vi "Voice Enhancement.vi"() -> ()   [LabVIEW 2023]
doc: "This example shows the application of linear Time Frequency Analysis VIs in online voice enhancement, or noise reduction in speech signals. Refer to the Online Noise Reduction example for more information about online noise reduction.\n\nThis example uses the TFA Online Gabor Transform VI to convert a speech signal into the time-frequency representation, sets the Gabor coefficients whose magnitude is smaller than a threshold to zero, and finally uses the TFA Online Gabor Expansion VI to reconstruct the enhanced speech signal. \n\n<b>Instructions:</b>\n1) Run this VI.\n2) Speak into the microphone in a noisy environment.\n3) Listen the enhanced voice by using the headset."
uses:
  <vilib>/sound2/lvsound2.llb/Sound Data Format.ctl
  <vilib>/sound2/lvsound2.llb/Sound Input Read (DBL).vi
  <vilib>/addons/Time Frequency Analysis/Transform.llb/TFA Online Gabor Transform (Real).vi
  <vilib>/addons/Time Frequency Analysis/Transform.llb/TFA Online Gabor Expansion (Real).vi
  <vilib>/sound2/lvsound2.llb/Sound Output Write (DBL Single).vi
  <vilib>/addons/_Advanced Signal Processing/NI_AdvSigProcTFA.lvlib
panel:
  out "aspt-left-top":bool
  in  "Replay?(F)":bool
  in  "Attenuation factor":dbl=0.2
  in  "reset":bool
  out "Enhanced Speech":dbl[](graph)
  out "Noise Speech":dbl[](graph)
  out "Enhanced Gabor Coefficients":dbl[][](graph)
  out "Magnitude of Gabor Coefficients":dbl[][](graph)
  in  "Enhance?":bool=TRUE
  in  "Noise level":dbl=1.2
  in  "Stop":bool
  # "Overview: Shows the application of linear Time Frequency Analysis VIs in online voice enhancement, or noise reduction in speech signals. Refer to the Online Noise Reduction example for more information about online noise reduction.\nRequirements: LabVIEW Full Development System, Advanced Signal Processing Toolkit, microphone\nInstructions: \n1. Run this VI.\n2. Speak into the microphone in a noisy environment.\n3. Listen the enhanced voice by using the headset.\n4. Click Stop to stop the VI."
  # "Time Domain"
  # "Processing in Joint Time-Frequency Domain"
  # "Time Domain"
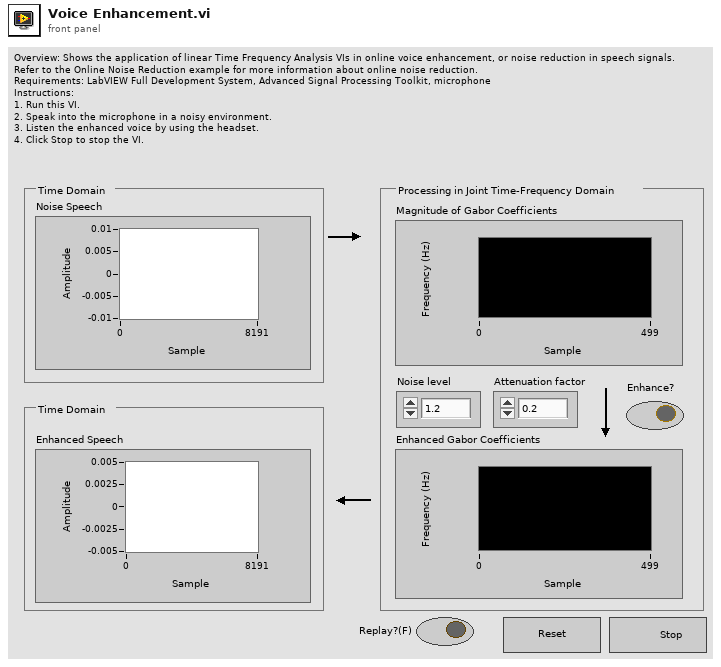
[diagram p1: front panel]
types:
  T1 = typedef "Sound Data Format.ctl" = cluster{"sample rate (S/s)":dbl, "number of channels":i32, "bits per sample":i32}
  T2 = typedef "Sound Input Task ID.ctl" = u32
  T3 = typedef "Sound Output Task ID.ctl" = u32
  T4 = cluster{"synthesis window":dbl[], "dM (time steps)":i32, "N (frequency bins)":i32}
  T5 = cluster{"analysis window":dbl[], "dM (time steps)":i32, "N (frequency bins)":i32}
  T6 = cluster{"frequency offset":dbl, "frequency multiplier":dbl}
  T7 = typedef "LVRangeTypeDef.ctl" = cluster{"Minimum":dbl, "Maximum":dbl, "Increment":dbl, "Minor Increment":dbl, "Start":dbl}
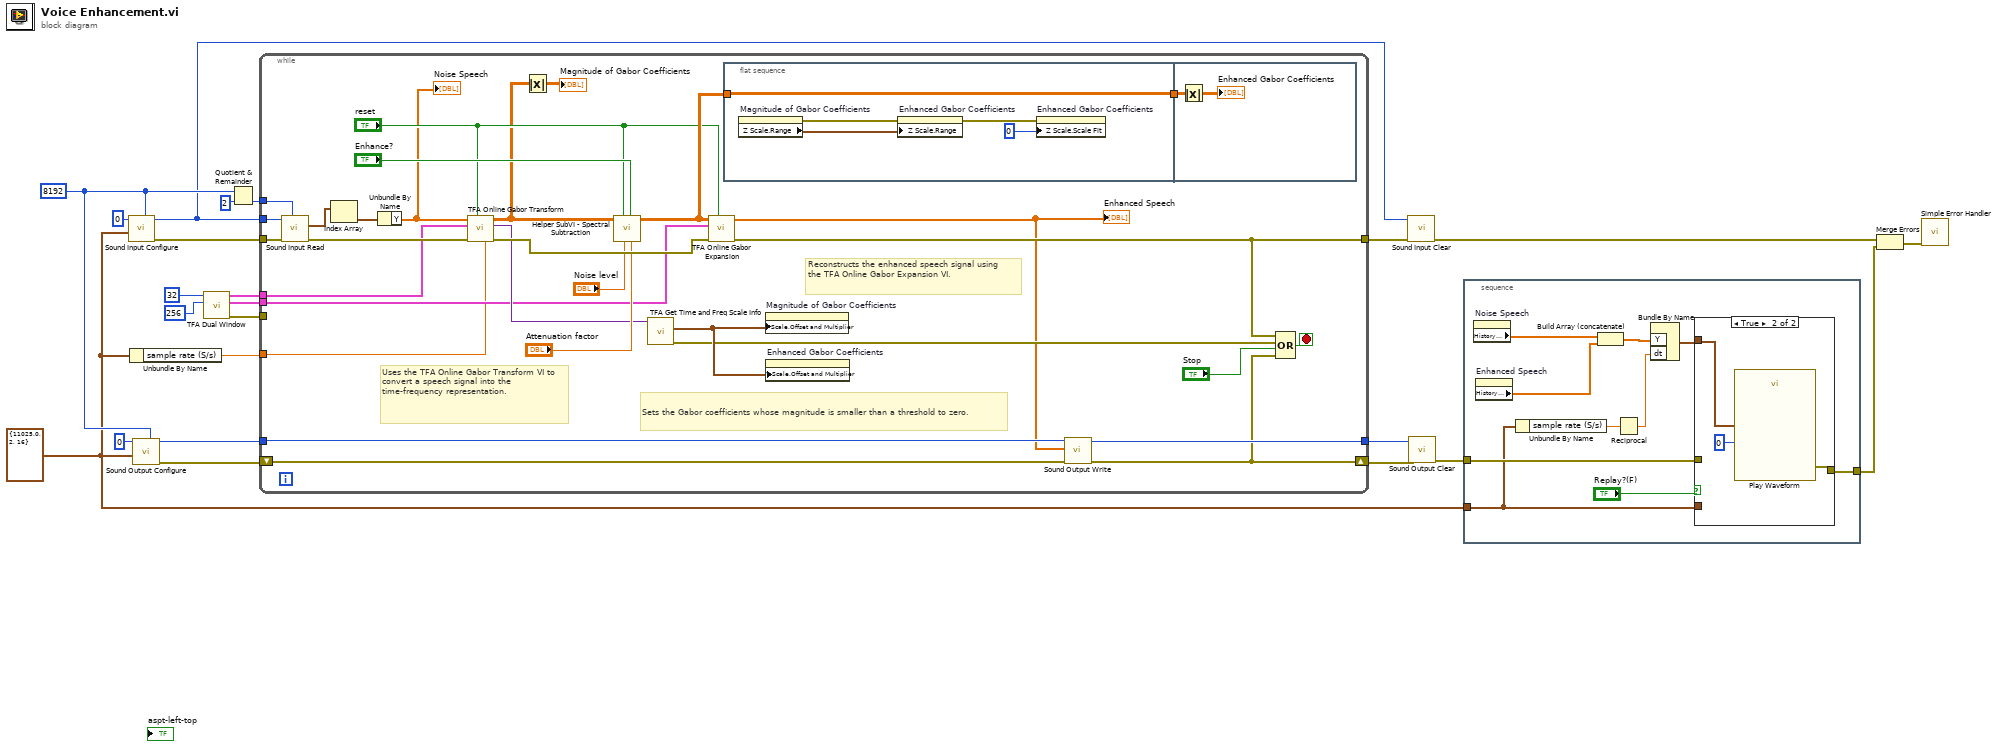
[diagram p0: block diagram]
diagram:
  w9 = 8192 ("number of samples/ch")
  w1 = T1 {"sample rate (S/s)"=11025.0, "number of channels"=2, "bits per sample"=16} ("sound format")
  n1 = call <vilib>:"Sound Input Configure.vi"("number of samples/ch"=w9, "sound format"=w1, "device ID"=u32 0 ("device (0)")) -> ("error out"=w11:errorcluster, "task ID"=w5:T2)  [unwired: 7 in]
  n2 = Unbundle By Name(w1) -> ("sample rate (S/s)"=w12:dbl)
  n3 = call <vilib>:"Sound Output Configure.vi"("number of samples/ch"=w9, "sound format"=w1, "device ID"=u32 0 ("device (0)")) -> ("error out"=w6:errorcluster, "task ID"=w7:T3)  [unwired: 7 in]
  n4 = call <vilib>:"TFA Dual Window.vi"("N (frequency bins)"=256 ("num of freq bins"), "dM (time steps)"=32 ("time interval")) -> ("error out"=w16:errorcluster, "synthesis info"=w17:T4, "analysis info"=w18:T5)  [unwired: 2 in, 5 out]
  n5 = Quotient & Remainder(x=w9, y=2) -> (floor(x/y)=w8:i32)  [unwired: 1 out]
  n6 = while {
    tunnel: w5 -> [w53]
    tunnel: w11 -> [w52]
    tunnel: [w33] -> w4
    tunnel: w7 -> [w29]
    tunnel: [w48] -> w3
    shift-right: [w32] -> w2
    shift-left: w6 -> [w28]
    tunnel: w18 -> [w44]
    tunnel: w17 -> [w41]
    tunnel: w12 -> [w39]
    tunnel: w16 -> [_]
    tunnel: w8 -> [w27]
    stop <- w37 stop-if-true
    # "Uses the TFA Online Gabor Transform VI to convert a speech signal into the time-frequency representation."
    # "Sets the Gabor coefficients whose magnitude is smaller than a threshold to zero."
    # "Reconstructs the enhanced speech signal using the TFA Online Gabor Expansion VI."
    n7 = call-poly <vilib>:"Sound Input Read.vi"("number of samples/ch"=w27, "error in (no error)"=w52, "task ID"=w53) -> ("error out"=w51:errorcluster, "data"=w30:waveform(dbl)[])  [unwired: 6 in, 1 out]
    n8 = Index Array(array=w30) -> (element=w26:waveform(dbl))  [unwired: 1 in]
    n9 = Unbundle By Name(w26) -> ("Y"=w25:dbl[])
    "Noise Speech" <- w25
    n10 = call-poly <vilib>:"TFA Online Gabor Transform.vi"("sampling rate"=w39, "reset? (F)"="reset", "error in (no error)"=w51, "transform info"=w44, "signal"=w25) -> ("error out"=w49:errorcluster, "scale info"=w43:variant, "Gabor coef"=w35:cdb[][])  [unwired: 4 out]
    n11 = Absolute Value(x=w35) -> (abs(x)=→"Magnitude of Gabor Coefficients":dbl[][])
    n12 = call "Helper SubVI - Spectral Subtraction.vi"("attenuation factor"="Attenuation factor", "Enhance?"="Enhance?", "noise level"="Noise level", "reset"="reset", "Gabor coefficients in"=w35) -> ("Gabor coefficients out"=w40:cdb[][])  [unwired: 6 out]
    n13 = call <vilib>:"TFA Get Time and Freq Scale Info.vi"("scale info"=w43) -> ("error out"=w31:errorcluster, "frequency info"=w42:T6)  [unwired: 1 in, 8 out]
    n14 = call-poly <vilib>:"TFA Online Gabor Expansion.vi"("reset? (F)"="reset", "error in (no error)"=w49, "expansion info"=w41, "Gabor coef"=w40) -> ("error out"=w33:errorcluster, "signal"=w24:dbl[])  [unwired: 6 out]
    "Enhanced Speech" <- w24
    n15 = flat-sequence {
      tunnel: w40 -> [w54]
      tunnel: [w54] -> w34
      tunnel: w34 -> [w59]
      frame #0 {
        n16 = property on="Magnitude of Gabor Coefficients" class="IntChart (strict)"() -> (error out=w56:errorcluster, "Z Scale.Range"=w58:T7)  [unwired: 2 in, 1 out]
        n17 = property on="Enhanced Gabor Coefficients" class="IntChart (strict)"(error in=w56, "Z Scale.Range"=w58) -> (error out=w55:errorcluster)  [unwired: 1 in, 1 out]
        n18 = property on="Enhanced Gabor Coefficients" class="IntChart (strict)"(error in=w55, "Z Scale.Scale Fit"=0) -> ()  [unwired: 1 in, 2 out]
      }
      frame #1 {
        n19 = Absolute Value(x=w59) -> (abs(x)=→"Enhanced Gabor Coefficients":dbl[][])
      }
    }
    n20 = property on="Magnitude of Gabor Coefficients" class="IntChart (strict)"("Y Scale.Offset and Multiplier"=w42) -> ()  [unwired: 2 in, 2 out]
    n21 = property on="Enhanced Gabor Coefficients" class="IntChart (strict)"("Y Scale.Offset and Multiplier"=w42) -> ()  [unwired: 2 in, 2 out]
    n22 = call-poly <vilib>:"Sound Output Write.vi"("error in (no error)"=w28, "data"=w24, "task ID"=w29) -> ("error out"=w32:errorcluster, "task ID out"=w48:T3)  [unwired: 7 in]
    n23 = Compound Arithmetic op=OR(w33, w31, "Stop", w32) -> (w37:bool)
  }
  n24 = call <vilib>:"Sound Input Clear.vi"("error in (no error)"=w4, "task ID"=w5) -> ("error out"=w15:errorcluster)  [unwired: 9 in]
  n25 = call <vilib>:"Sound Output Clear.vi"("error in (no error)"=w2, "task ID"=w3) -> ("error out"=w21:errorcluster)  [unwired: 9 in]
  n26 = stacked-sequence {
    tunnel: w21 -> [w70]
    tunnel: [w68] -> w14
    tunnel: w1 -> [w64]
    frame #0 {
      n27 = property on="Noise Speech" class="WFChart (strict)"() -> ("History Data"=w67:dbl[])  [unwired: 2 in, 2 out]
      n28 = property on="Enhanced Speech" class="WFChart (strict)"() -> ("History Data"=w66:dbl[])  [unwired: 2 in, 2 out]
      n29 = Unbundle By Name(w64) -> ("sample rate (S/s)"=w63:dbl)
      n30 = Build Array (concatenate)(w67, w66) -> (w65:dbl[])
      n31 = Reciprocal(x=w63) -> (1/x=w62:dbl)
      n32 = Bundle By Name("Y"=w65, "dt"=w62) -> (w61:waveform(dbl))  [unwired: 1 in]
      n33 = case shown="True" "Replay?(F)" {
        tunnel: w70 -> [w71 _]
        tunnel: w64 -> [_ _]
        tunnel: [w71 w73] -> w68
        tunnel: w61 -> [_ w72]
        frame False {
        }
        frame True {
          n34 = call "Play Waveform"("Device"=u32 0, "Data"=w72) -> ("error out"=w73:errorcluster)  [unwired: 17 in]
        }
      }
    }
  }
  n35 = Merge Errors(w15, w14) -> (w13:errorcluster)
  n36 = call <vilib>:"Simple Error Handler.vi"("error in (no error)"=w13) -> ()  [unwired: 4 in, 5 out]
